vi "AI-Channel Data to String Conversion.vi"(0 "All Object Ref":refnum<vi>[](array[refnum]), 2 "XML String In":string, 5 "All Object Label":string[](array[string]), 9 "Channel Types'":cluster{"Channel Type":T1, "Sub-Type":T2}, 13 "Write to Ctrl (F)":bool) -> (4 "XML String Out":string)   [LabVIEW 2021, in "Configuration.lvlib"]
doc: "<b>Note:</b> This VI was modified by the <b>Validate DQMH Module</b> tool to turn off automatic error handling."
uses:
  Configuration.lvlib
  Config-Channel Type.ctl
  Channel Sub-Type.ctl
  AI-Voltage Channel Data's.ctl
  AI-Current Channel Data's--Cluster.ctl
  AI-Thermocouple Data's.ctl
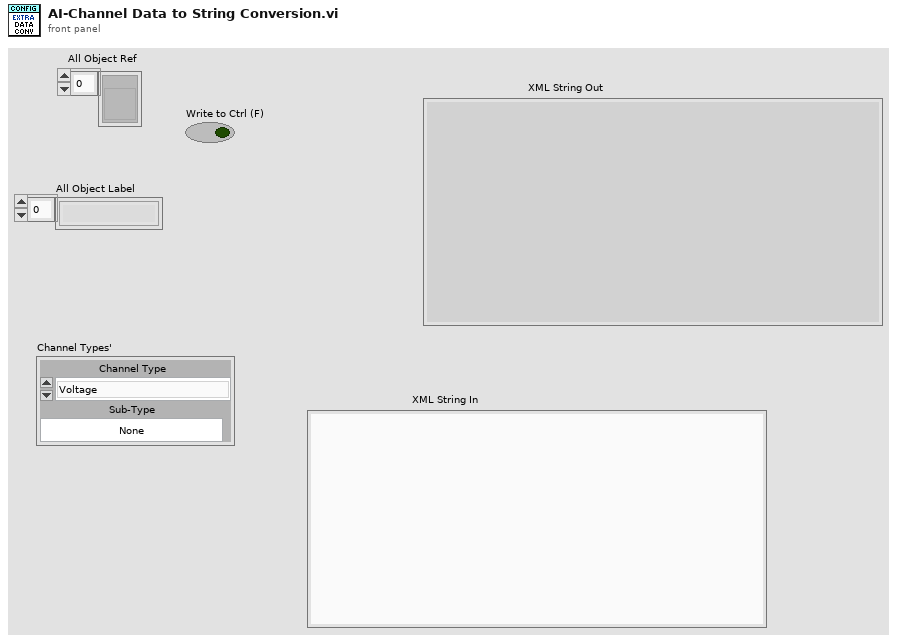
[diagram p1: front panel]
types:
  T1 = typedef "Configuration.lvlib/Config-Channel Type.ctl" = enum16{"Voltage", "Current", "Thermocouple", "Acclerometer"}
  T2 = typedef "Configuration.lvlib/Channel Sub-Type.ctl" = enum16{"None", "Pressure", "Force"}
  T3 = typedef "Configuration.lvlib/AI-Voltage Channel Data's.ctl" = cluster{"input terminal configuration":i32, "maximum value":dbl, "minimum value":dbl, "units":i32}
  T4 = typedef "Configuration.lvlib/AI-Current Channel Data's--Cluster.ctl" = cluster{"maximum value":dbl, "minimum value":dbl, "input terminal configuration":i32, "external shunt resistor value":dbl, "units":i32, "shunt resistor location":i32}
  T5 = typedef "Configuration.lvlib/AI-Thermocouple Data's.ctl" = cluster{"thermocouple type":i32, "maximum value":dbl, "minimum value":dbl, "units":i32}
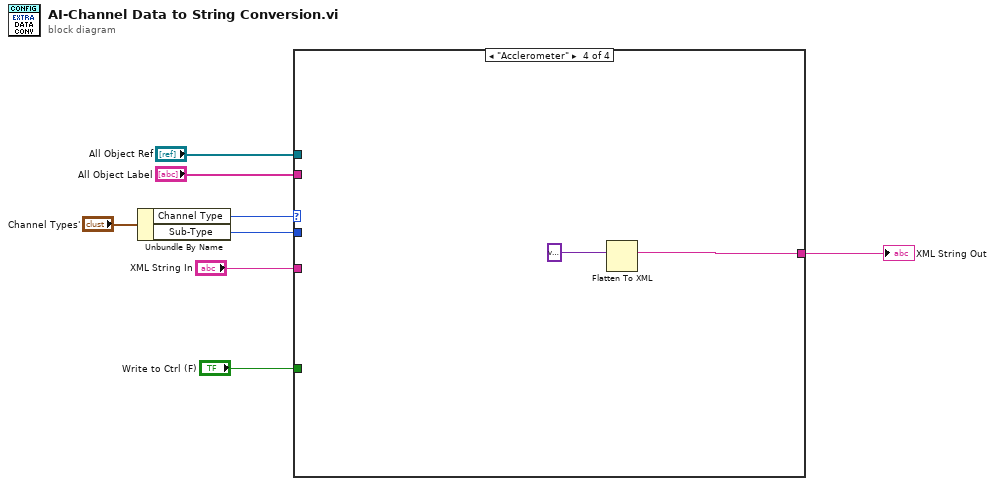
[diagram p0: block diagram]
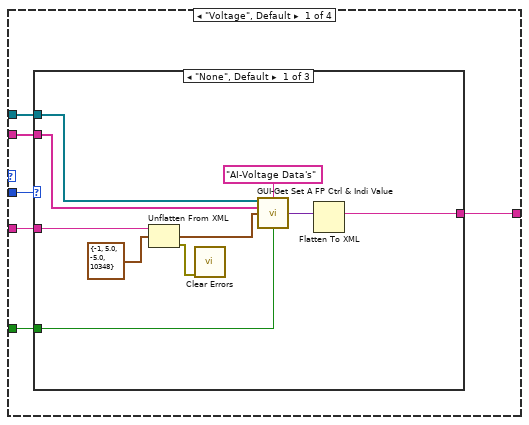
[diagram p2: hidden frame]
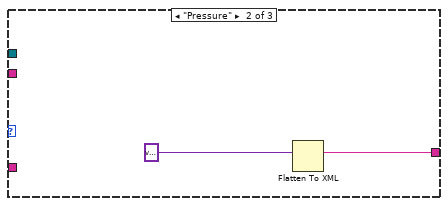
[diagram p3: hidden frame]
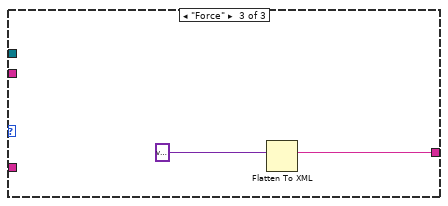
[diagram p4: hidden frame]
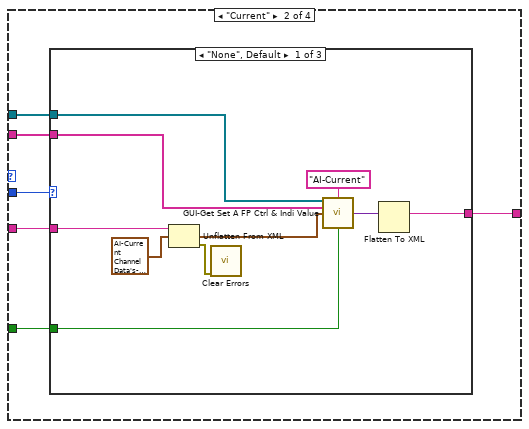
[diagram p5: hidden frame]
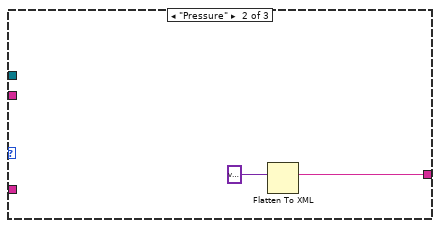
[diagram p6: hidden frame]
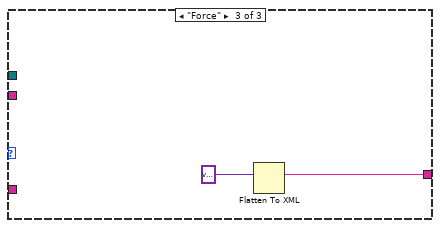
[diagram p7: hidden frame]
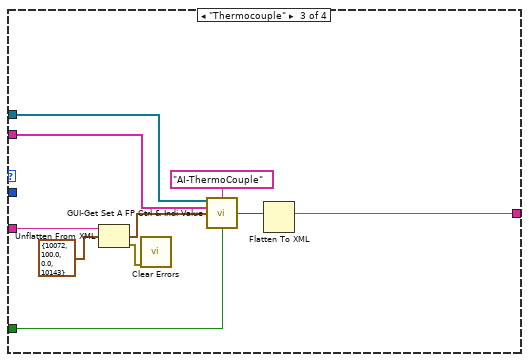
[diagram p8: hidden frame]
diagram:
  n1 = Unbundle By Name("Channel Types'") -> ("Channel Type"=w7:T1, "Sub-Type"=w6:T2)
  n2 = case shown="\"Acclerometer\"" w7 {
    tunnel: w6 -> [w14 w33 _ _]
    tunnel: [w13 w34 w54 w59] -> w5
    tunnel: "All Object Ref" -> [w12 w32 w57 _]
    tunnel: "All Object Label" -> [w11 w31 w56 _]
    tunnel: "XML String In" -> [w10 w30 w51 _]
    tunnel: "Write to Ctrl (F)" -> [w9 w29 w49 _]
    frame "Voltage", Default {
      n3 = case shown="\"None\", Default" w14 {
        tunnel: [w20 w25 w27] -> w13
        tunnel: w12 -> [w23 _ _]
        tunnel: w11 -> [w22 _ _]
        tunnel: w10 -> [w19 _ _]
        tunnel: w9 -> [w18 _ _]
        frame "None", Default {
          n4 = Unflatten From XML(xml string=w19, type=T3 {"input terminal configuration"=-1, "maximum value"=5.0, "minimum value"=-5.0, "units"=10348} ("AI-Voltage Data's")) -> (value=w16:T3, error out=w15:errorcluster)  [unwired: 1 in]
          n5 = call <vilib>:"Clear Errors.vi"("error in (no error)"=w15) -> ()  [unwired: 5 in, 2 out]
          n6 = call "GUI-Get Set A FP Ctrl & Indi Value.vi"("All Object Ref"=w23, "Label"="AI-Voltage Data's" ("Label In"), "All Object Label"=w22, "Ctrl Value In"=w16, "Set(F)"=w18) -> ("Ctrl Value Out"=w21:variant)  [unwired: 7 in, 3 out]
          n7 = Flatten To XML(6:w21) -> (2:w20:string)
        }
        frame "Pressure" {
          n8 = Flatten To XML(6:variant ("Variant")) -> (2:w25:string)
        }
        frame "Force" {
          n9 = Flatten To XML(6:variant ("Variant")) -> (2:w27:string)
        }
      }
    }
    frame "Current" {
      n10 = case shown="\"None\", Default" w33 {
        tunnel: [w40 w45 w47] -> w34
        tunnel: w32 -> [w44 _ _]
        tunnel: w31 -> [w43 _ _]
        tunnel: w30 -> [w38 _ _]
        tunnel: w29 -> [w35 _ _]
        frame "None", Default {
          n11 = Unflatten From XML(xml string=w38, type=T4 {"maximum value"=0.01, "minimum value"=-0.01, "input terminal configuration"=-1, "external shunt resistor value"=249.0, "units"=10342, "shunt resistor location"=-1} ("AI-Current")) -> (value=w37:T4, error out=w39:errorcluster)  [unwired: 1 in]
          n12 = call <vilib>:"Clear Errors.vi"("error in (no error)"=w39) -> ()  [unwired: 5 in, 2 out]
          n13 = call "GUI-Get Set A FP Ctrl & Indi Value.vi"("All Object Ref"=w44, "Label"="AI-Current" ("Label In"), "All Object Label"=w43, "Ctrl Value In"=w37, "Set(F)"=w35) -> ("Ctrl Value Out"=w41:variant)  [unwired: 7 in, 3 out]
          n14 = Flatten To XML(6:w41) -> (2:w40:string)
        }
        frame "Pressure" {
          n15 = Flatten To XML(6:variant ("Variant")) -> (2:w45:string)
        }
        frame "Force" {
          n16 = Flatten To XML(6:variant ("Variant")) -> (2:w47:string)
        }
      }
    }
    frame "Thermocouple" {
      n17 = Unflatten From XML(xml string=w51, type=T5 {"thermocouple type"=10072, "maximum value"=100.0, "minimum value"=0.0, "units"=10143} ("AI-ThermoCouple")) -> (value=w50:T5, error out=w53:errorcluster)  [unwired: 1 in]
      n18 = call <vilib>:"Clear Errors.vi"("error in (no error)"=w53) -> ()  [unwired: 5 in, 2 out]
      n19 = call "GUI-Get Set A FP Ctrl & Indi Value.vi"("All Object Ref"=w57, "Label"="AI-ThermoCouple" ("Label In"), "All Object Label"=w56, "Ctrl Value In"=w50, "Set(F)"=w49) -> ("Ctrl Value Out"=w55:variant)  [unwired: 7 in, 3 out]
      n20 = Flatten To XML(6:w55) -> (2:w54:string)
    }
    frame "Acclerometer" {
      n21 = Flatten To XML(6:variant ("Variant")) -> (2:w59:string)
    }
  }
  "XML String Out" <- w5
